vi "Ring Buffer Online Far.vi"(9 "Index":i32, 10 "Profiles to Average":i32, 11 "Input Array":dbl[](array[numeric])) -> (1 "AvgArray":dbl[](array[numeric]), 3 "RingBufferOut":dbl[][](array[numeric]))   [LabVIEW 2012]
panel:
  out "RingArraySize":dbl[](array[numeric])
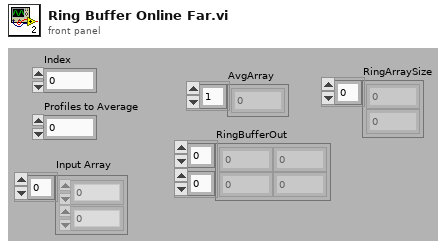
[diagram p1: front panel]
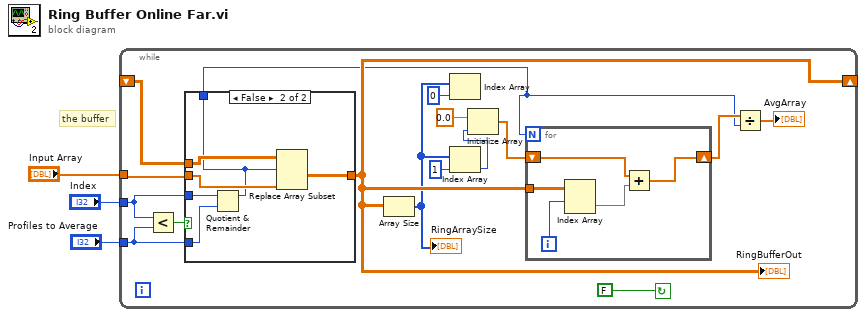
[diagram p0: block diagram]
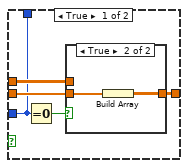
[diagram p2: hidden frame]
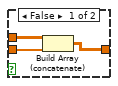
[diagram p3: hidden frame]
diagram:
  # "the buffer"
  n1 = while {
    shift-right: [w11] -> _
    shift-left: _ -> [w14]
    tunnel: "Profiles to Average" -> [w17]
    tunnel: "Index" -> [w16]
    tunnel: "Input Array" -> [w15]
    stop <- FALSE ("stop") continue-if-true
    n2 = Less?(x=w16, y=w17) -> (x < y?=w18:bool)
    n3 = case shown="False" w18 {
      tunnel: w16 -> [w25 w40]
      tunnel: [w26 w36] -> w11
      tunnel: w17 -> [_ w39]
      tunnel: w15 -> [w27 w37]
      tunnel: w14 -> [w28 w38]
      tunnel: [w25 w35] -> w4
      frame True {
        n4 = Equal To 0?(x=w25) -> (x = 0?=w29:bool)
        n5 = case shown="True" w29 {
          tunnel: [w30 w34] -> w26
          tunnel: w28 -> [w32 _]
          tunnel: w27 -> [w31 w33]
          frame False {
            n6 = Build Array (concatenate)(w32, w31) -> (w30:dbl[][])
          }
          frame True {
            n7 = Build Array(w33) -> (w34:dbl[][])
          }
        }
      }
      frame False {
        n8 = Quotient & Remainder(x=w40, y=w39) -> (x-y*floor(x/y)=w35:i32)  [unwired: 1 out]
        n9 = Replace Array Subset(array=w38, new element=w37, index (row)=w35) -> (w36:dbl[][])  [unwired: 1 in]
      }
    }
    "RingBufferOut" <- w11
    n10 = Array Size(array=w11) -> (size(s)=w5:i32[])
    "RingArraySize" <- w5
    n11 = Index Array(array=w5, index=0) -> ()  [unwired: 1 out]
    n12 = Index Array(array=w5, index=1) -> (element=w10:i32)
    n13 = Initialize Array(0.0, w10) -> (w8:dbl[])
    n14 = for {
      N: w4 -> [_]
      tunnel: w11 -> [w24]
      shift-right: [w20] -> w7
      shift-left: w8 -> [w21]
      i -> [w23]
      n15 = Index Array(array=w24, index (row)=w23) -> (element=w22:dbl[])  [unwired: 1 in]
      n16 = Add(x=w21, y=w22) -> (x+y=w20:dbl[])
    }
    n17 = Divide(x=w7, y=w4) -> (x/y=→"AvgArray":dbl[])
  }
